vi "Status Manager Close.vi"(8 "error in":errorcluster, 11 "Status References":T1[](array[typedef])) -> (0 "error out":errorcluster)   [LabVIEW 2021, in "Status.lvlib"]
uses:
  Status.lvlib
  Ctl/control.ctl
  Ctl/State.ctl
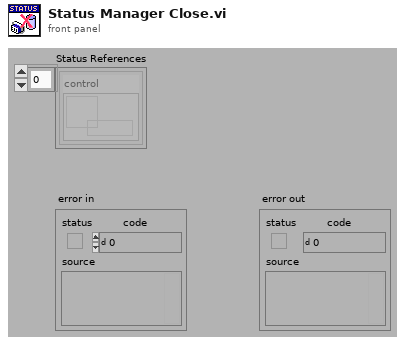
[diagram p1: front panel]
types:
  T1 = typedef "Status.lvlib/control.ctl" = cluster{"control":refnum<data-value>}
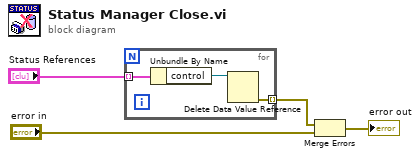
[diagram p0: block diagram]
diagram:
  n1 = for {
    tunnel: [w7] -> w3 mode=indexing
    tunnel: "Status References" -> [w5] mode=indexing
    n2 = Unbundle By Name(w5) -> ("control"=w6:refnum<data-value>)
    n3 = Delete Data Value Reference(data value reference=w6) -> (error out=w7:errorcluster)  [unwired: 1 in, 1 out]
  }
  n4 = Merge Errors(w3, "error in") -> (→"error out":errorcluster)
